vi "Generate tracks.vi"(8 "error in (no error)":errorcluster, 10 "Hits to display":T2, 11 "Event display in":refnum<vi>) -> (0 "error out":errorcluster, 3 "Event display out":refnum<vi>)   [LabVIEW 2016]
uses:
  Typedefs/Coincidence.ctl
  <vilib>/picture/3D Picture Control/Object/Create Object (name).vi
  <vilib>/picture/3D Picture Control/NI_3D Picture Control.lvlib
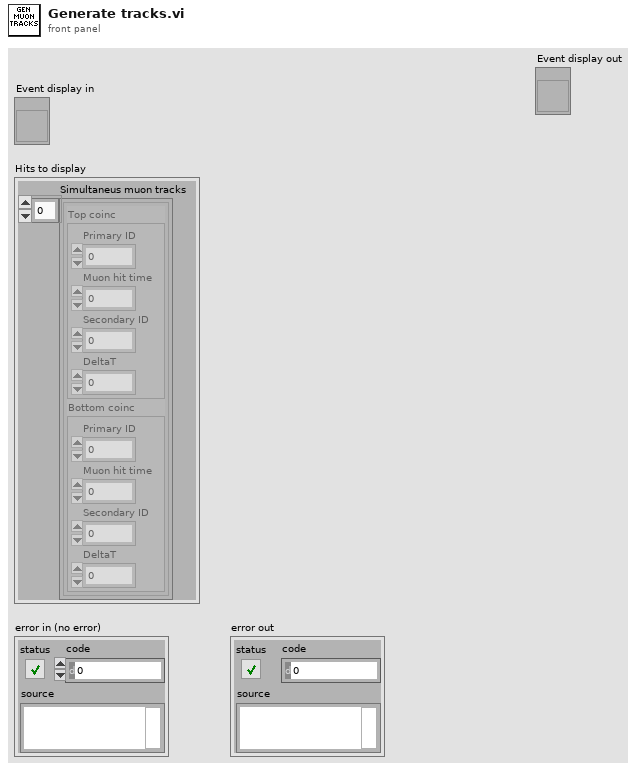
[diagram p1: front panel]
types:
  T1 = typedef "Coincidence.ctl" = cluster{"Primary ID":i8, "Muon hit time":u64, "Secondary ID":i8, "DeltaT":i32}
  T2 = cluster{"Simultaneus muon tracks":cluster{"Top coinc":T1, "Bottom coinc":T1}[]}
  T3 = cluster{"Red":sgl, "Green":sgl, "Blue":sgl, "Alpha":sgl}
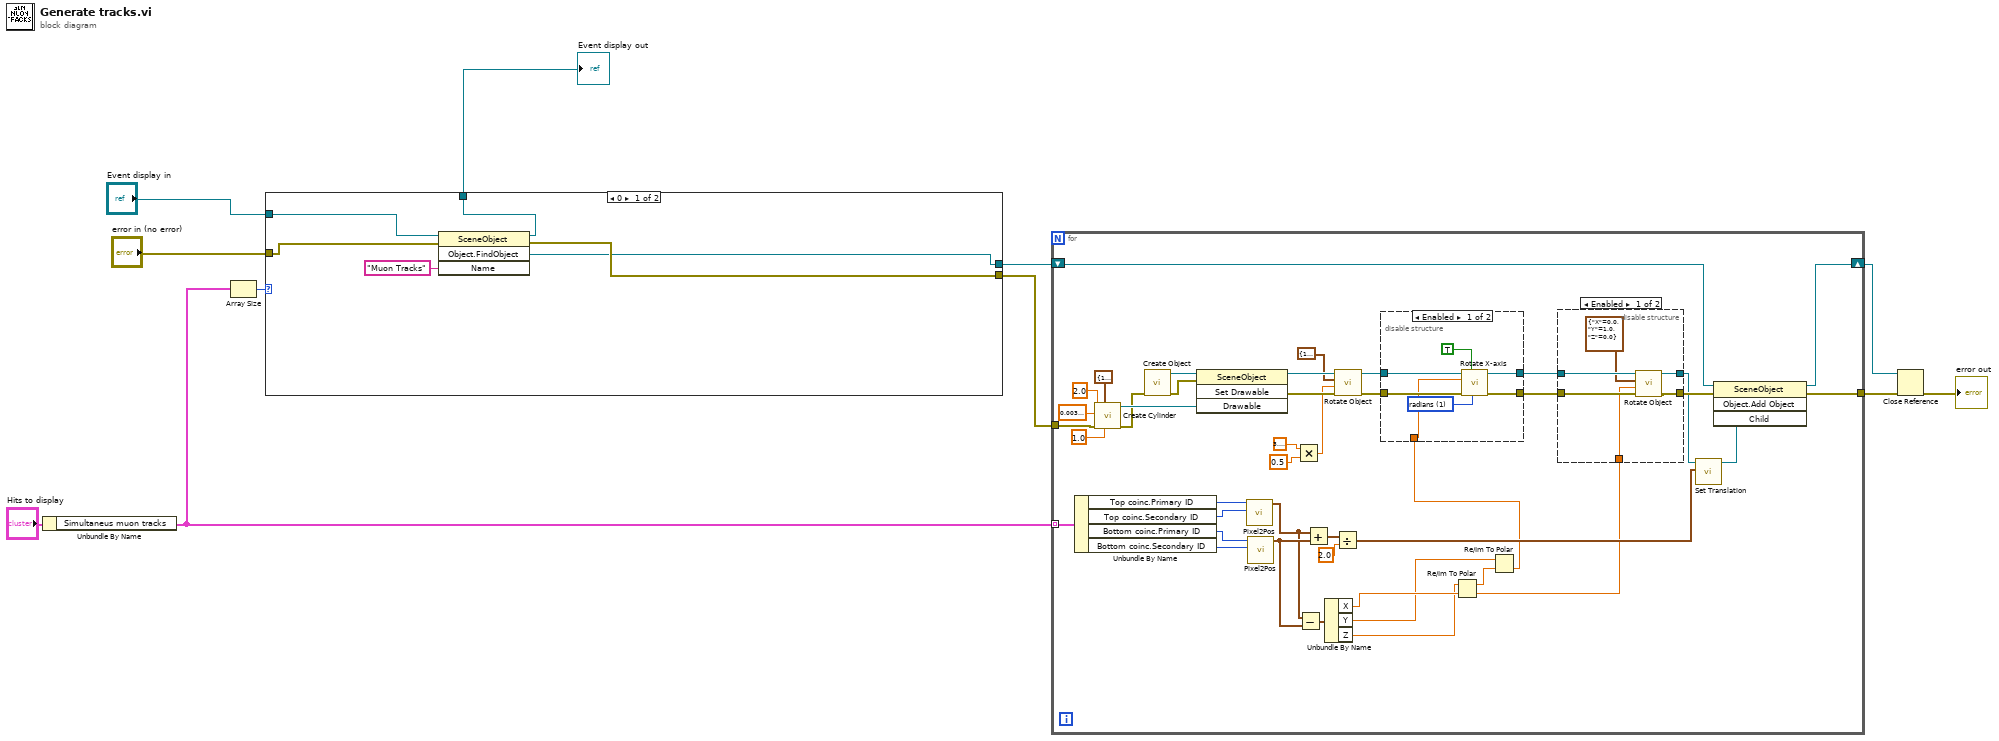
[diagram p0: block diagram]
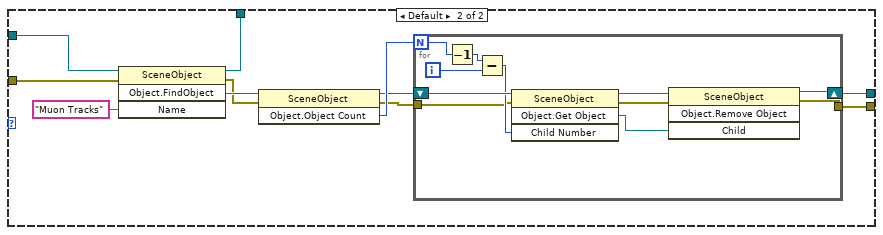
[diagram p2: hidden frame]
diagram:
  n1 = Unbundle By Name("Hits to display") -> ("Simultaneus muon tracks"=w1:cluster{"Top coinc":T1, "Bottom coinc":T1}[])
  n2 = Array Size(array=w1) -> (size(s)=w2:i32)
  n3 = case shown="0" w2 {
    tunnel: "Event display in" -> [w15 w28]
    tunnel: [w12 w23] -> w10
    tunnel: "error in (no error)" -> [w16 w22]
    tunnel: [w13 w19] -> w8
    tunnel: [w14 w18] -> w7
    frame 0 {
      n4 = invoke class="SceneObject" method="Object.FindObject"(reference=w15, error in=w16, "Name"="Muon Tracks") -> (reference out=w14:refnum<vi>, error out=w13:errorcluster, "FindObject"=w12:refnum<vi>)  [unwired: 1 in, 1 out]
    }
    frame Default {
      n5 = invoke class="SceneObject" method="Object.FindObject"(reference=w28, error in=w22, "Name"="Muon Tracks") -> (reference out=w18:refnum<vi>, error out=w21:errorcluster, "FindObject"=w26:refnum<vi>)  [unwired: 1 in, 1 out]
      n6 = invoke class="SceneObject" method="Object.Object Count"(reference=w26, error in=w21) -> (reference out=w24:refnum<vi>, error out=w20:errorcluster, "Child Count"=w25:i32)  [unwired: 1 in]
      n7 = for {
        N: w25 -> [w37]
        shift-right: [w31] -> w23
        shift-left: w24 -> [w39]
        tunnel: w20 -> [w30]
        tunnel: [w29] -> w19
        i -> [w38]
        n8 = Decrement(x=w37) -> (x-1=w36:i32)
        n9 = Subtract(x=w36, y=w38) -> (x-y=w35:i32)
        n10 = invoke class="SceneObject" method="Object.Get Object"(reference=w39, error in=w30, "Child Number"=w35) -> (reference out=w34:refnum<vi>, error out=w33:errorcluster, "Get Child"=w32:refnum<vi>)  [unwired: 1 in, 1 out]
        n11 = invoke class="SceneObject" method="Object.Remove Object"(reference=w34, error in=w33, "Child"=w32) -> (reference out=w31:refnum<vi>, error out=w29:errorcluster)  [unwired: 1 in, 2 out]
      }
    }
  }
  "Event display out" <- w7
  n12 = for {
    shift-right: [w68] -> w6
    shift-left: w10 -> [w69]
    tunnel: w8 -> [w67]
    tunnel: w1 -> [w66] mode=indexing
    tunnel: [w65] -> w5
    n13 = Unbundle By Name(w66) -> ("Top coinc.Primary ID"=w72:i8, "Top coinc.Secondary ID"=w73:i8, "Bottom coinc.Primary ID"=w74:i8, "Bottom coinc.Secondary ID"=w75:i8)
    n14 = call <vilib>:"Create Cylinder.vi"("Detail"=sgl 1.0, "Color"=T3 {"Red"=1.0, "Green"=1.0, "Blue"=0.0, "Alpha"=1.0}, "error in (no error)"=w67, "Radius"=sgl 0.003, "Height"=sgl 2.0) -> ("error out"=w70:errorcluster, "New Cylinder Refnum"=w81:refnum<vi>)  [unwired: 5 in]
    n15 = call-poly <vilib>:"Create Object.vi"("error in (no error)"=w70) -> ("error out"=w71:errorcluster, "Scene:New Object"=w80:refnum<vi>)  [unwired: 9 in]
    n16 = invoke class="SceneObject" method="Set Drawable"(reference=w80, error in=w71, "Drawable"=w81) -> (reference out=w58:refnum<vi>, error out=w57:errorcluster)  [unwired: 1 in, 2 out]
    n17 = call "Pixel2Pos.vi"("Secondary"=w73, "Primary"=w72) -> ("Position (m)"=w54:cluster{"X":dbl, "\nY":dbl, "\nZ":dbl})  [unwired: 9 in]
    n18 = call "Pixel2Pos.vi"("Secondary"=w75, "Primary"=w74) -> ("Position (m)"=w60:cluster{"X":dbl, "\nY":dbl, "\nZ":dbl})  [unwired: 9 in]
    n19 = Multiply(x=3.141592653589793, y=0.5) -> (x*y=w55:dbl)
    n20 = Subtract(x=w54, y=w60) -> (x-y=w59:cluster{"X":dbl, "\nY":dbl, "\nZ":dbl})
    n21 = Add(x=w54, y=w60) -> (x+y=w62:cluster{"X":dbl, "\nY":dbl, "\nZ":dbl})
    n22 = Unbundle By Name(w59) -> ("X"=w44:dbl, "Y"=w43:dbl, "Z"=w42:dbl)
    n23 = Divide(x=w62, y=2.0) -> (x/y=w50:cluster{"X":dbl, "\nY":dbl, "\nZ":dbl})
    n24 = call <vilib>:"Rotate Object.vi"("error in (no error)"=w57, "Angle"=w55, "Axis"=cluster{"X":sgl, "Y":sgl, "Z":sgl} {"X"=1.0, "Y"=0.0, "Z"=0.0}, "Scene.Object In"=w58) -> ("error out"=w52:errorcluster, "Scene.Object Out"=w53:refnum<vi>)  [unwired: 6 in]
    n25 = Re/Im To Polar(2:w44, 3:w42) -> (0:w41:dbl, 1:w45:dbl)
    n26 = Re/Im To Polar(2:w45, 3:w43) -> (0:w40:dbl)  [unwired: 1 out]
    n27 = disable-structure shown="Enabled" {
      disable-tunnel: w53 -> [w95 w97]
      disable-tunnel: w40 -> [w90 _]
      disable-tunnel: [w94 w97] -> w48
      disable-tunnel: w52 -> [w93 w96]
      disable-tunnel: [w92 w96] -> w49
      frame Enabled {
        w89 = u16 1 items=["degree", "radians"] ("angle unit")
        n28 = call <vilib>:"Rotate X-axis.vi"("angle unit"=w89, "Relative?"=TRUE, "error in (no error)"=w93, "angle"=w90, "Scene Object In"=w95) -> ("error out"=w92:errorcluster, "Scene Object Out"=w94:refnum<vi>)  [unwired: 5 in]
      }
      frame Disabled {
      }
    }
    n29 = disable-structure shown="Enabled" {
      disable-tunnel: w49 -> [w87 _]
      disable-tunnel: w48 -> [w86 w88]
      disable-tunnel: [w85 _] -> w47
      disable-tunnel: [w84 w88] -> w46
      disable-tunnel: w41 -> [w83 _]
      frame Enabled {
        n30 = call <vilib>:"Rotate Object.vi"("error in (no error)"=w87, "Angle"=w83, "Axis"=cluster{"X":sgl, "Y":sgl, "Z":sgl} {"X"=0.0, "Y"=1.0, "Z"=0.0}, "Scene.Object In"=w86) -> ("error out"=w85:errorcluster, "Scene.Object Out"=w84:refnum<vi>)  [unwired: 6 in]
      }
      frame Disabled {
      }
    }
    n31 = call <vilib>:"Set Translation.vi"("Translation"=w50, "Scene Object"=w46) -> ("Translated Object"=w51:refnum<vi>)  [unwired: 8 in, 1 out]
    n32 = invoke class="SceneObject" method="Object.Add Object"(reference=w69, error in=w47, "Child"=w51) -> (reference out=w68:refnum<vi>, error out=w65:errorcluster)  [unwired: 1 in, 2 out]
  }
  n33 = Close Reference(reference=w6, error in (no error)=w5) -> (error out=→"error out":errorcluster)
